vi "Display.vi"(8 "error in":errorcluster, 11 "Custom - Two Button in":refnum<class "Gif - Two Button.lvclass">) -> (0 "error out":errorcluster, 3 "Custom - Two Button out":refnum<class "Gif - Two Button.lvclass">)   [LabVIEW 2021, in "Gif - Two Button.lvclass"]
doc: "This VI will display a custom image to the user along with their message and buttons for pos/neg choice\n\n<b>Code Developed By:</b>\nDaniel Coons\nTechnology Service Corporation\n1983 S Liberty Drive\nBloomington, IN 47403\nPhone: 812 558-7100\ndaniel.coons@tsc.com\nwww.tsc.com/atcs"
uses:
  Gif - Two Button.lvclass
  C:/Program Files/National Instruments/LabVIEW 2024/vi.lib/addons/_TSC/TSC Pop-Up/Popup/Popup.lvclass
  C:/Development/tsc-pop-up-gif/GIF Parent.lvclass
  <vilib>/Utility/miscctls.llb/LVPositionTypeDef.ctl
  Gif - Two Button.lvclass/Gif - Two Button.ctl
  <vilib>/addons/_TSC/TSC Pop-Up/Popup/Popup.lvclass/Popup.ctl
  GIF Parent.lvclass/GIF Parent.ctl
  <vilib>/addons/_TSC/TSC Pop-Up/Popup/Data Member Access/Read Theme.vi
  Read Delays.vi
  Read Gif Images.vi
  <vilib>/addons/_TSC/TSC Pop-Up/Theme/Theme.lvclass
  <vilib>/addons/_TSC/TSC Pop-Up/Popup/Popup.lvclass
  user32.dll
panel:
  in  "closer":bool
  out "header":bool
  in  "n-choice":bool
  in  "y-choice":bool
  out "2D Picture":picture
  out "Message":string
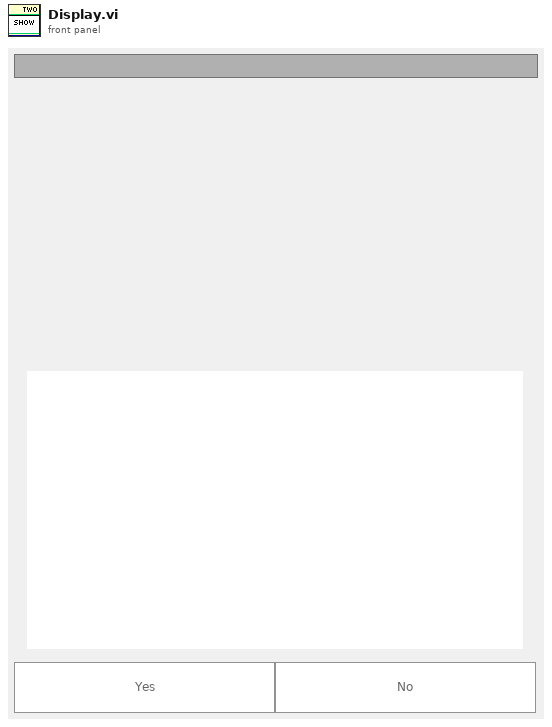
[diagram p1: front panel]
types:
  T1 = typedef "LVPositionTypeDef.ctl" = cluster{"Left":i32, "Top":i32}
  T2 = typedef "LVPoint32TypeDef.ctl" = cluster{"Horizontal":i32, "Vertical":i32}
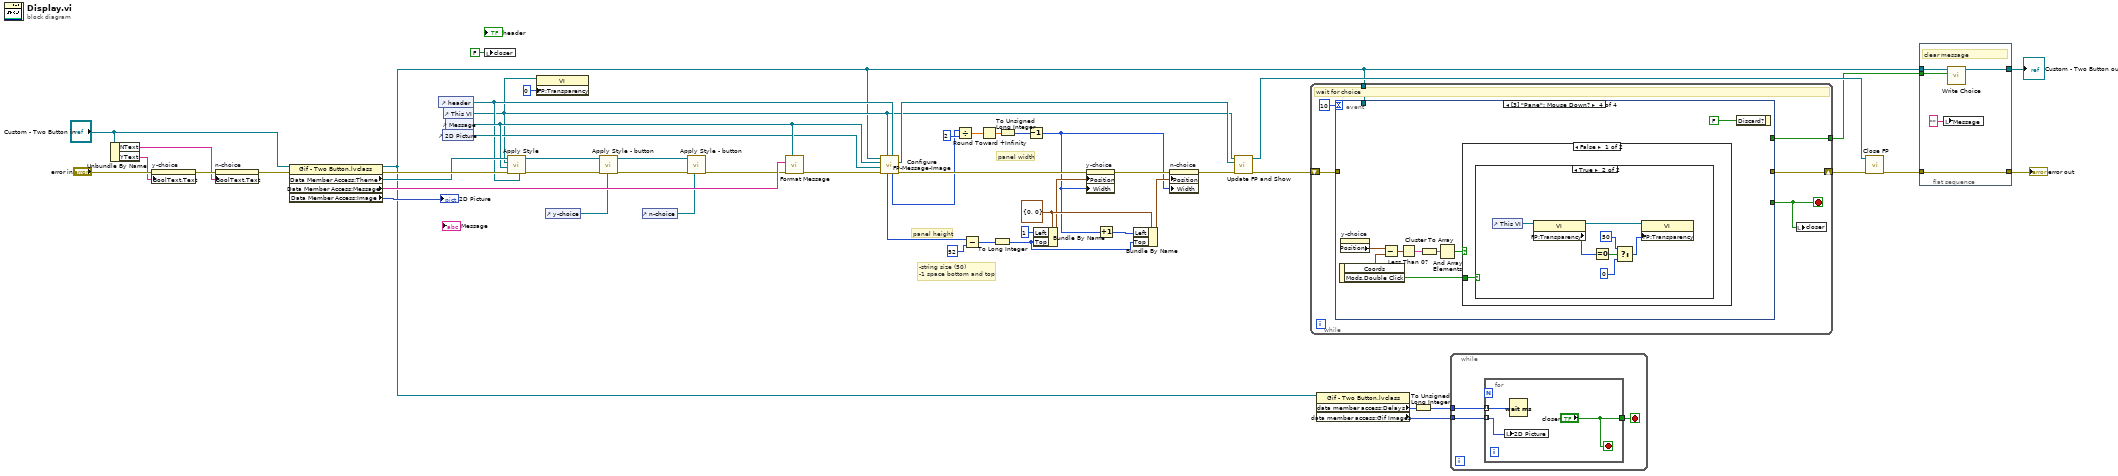
[diagram p0: block diagram]
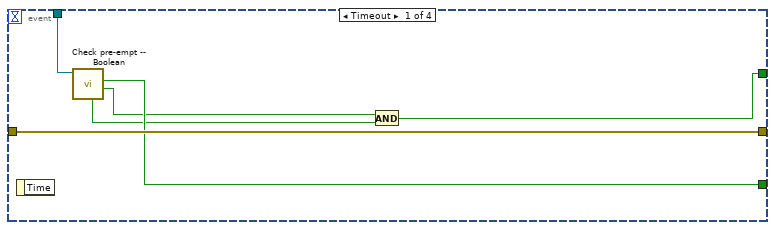
[diagram p2: hidden frame]
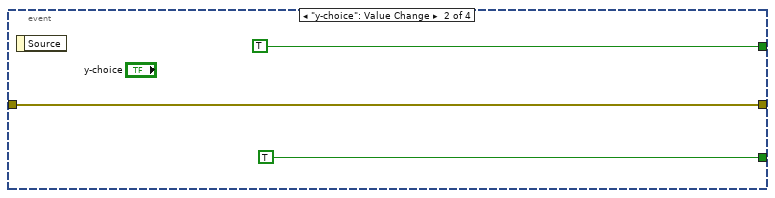
[diagram p3: hidden frame]
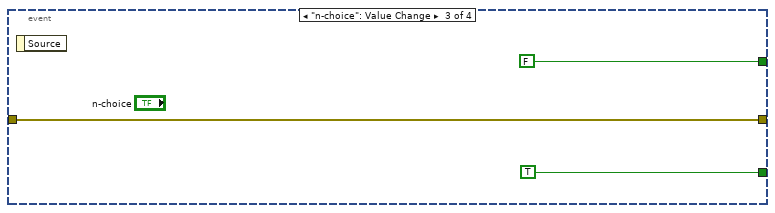
[diagram p4: hidden frame]
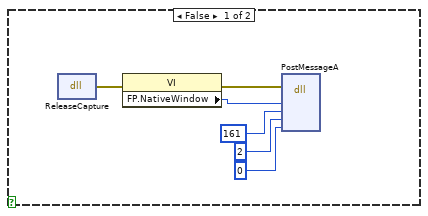
[diagram p5: hidden frame]
diagram:
  w41 = T1 {"Left"=0, "Top"=0} ("Position")
  # "-string size (50)\n-1 space bottom and top"
  # "panel width"
  # "panel height"
  n1 = Unbundle By Name("Custom - Two Button in") -> ("NText"=w43:string, "YText"=w46:string)
  n2 = property on="y-choice" class="Bool"(error in="error in", "BoolText.Text"=w46) -> (error out=w45:errorcluster)  [unwired: 1 in, 1 out]
  n3 = property on="n-choice" class="Bool"(error in=w45, "BoolText.Text"=w43) -> (error out=w44:errorcluster)  [unwired: 1 in, 1 out]
  n4 = property class="Gif - Two Button.lvclass"(reference="Custom - Two Button in", error in=w44) -> (reference out=w1:refnum<class "Gif - Two Button.lvclass">, error out=w28:errorcluster, "Data Member Access:Theme"=w26:refnum<class "Theme.lvclass">, "Data Member Access:Message"=w25:string, "Data Member Access:Image"=→"2D Picture":picture)
  n5 = control-ref of="header"() -> (w14:refnum<vi>)
  n6 = control-ref of="2D Picture"() -> (w15:refnum<vi>)
  n7 = control-ref of="This VI"() -> (w7:refnum<vi>)
  n8 = control-ref of="Message"() -> (w16:refnum<vi>)
  n9 = local write "closer"(FALSE ("closer")) -> ()
  n10 = call <vilib>:"Apply Style.vi"("header ref"=w14, "error in (no error)"=w28, "message ref"=w16, "pop up ref"=w7, "Theme in"=w26) -> ("error out"=w27:errorcluster, "Theme out"=w20:refnum<class "Theme.lvclass">)  [unwired: 5 in]
  n11 = property class="VI"(reference=w7, "FP:Transparency"=u8 0 ("Front Panel Window:Transparency")) -> ()  [unwired: 1 in, 2 out]
  n12 = control-ref of="y-choice"() -> (w21:refnum<vi>)
  n13 = call <vilib>:"Apply Style - button.vi"("button ref"=w21, "error in (no error)"=w27, "Theme in"=w20) -> ("error out"=w23:errorcluster, "Theme out"=w18:refnum<class "Theme.lvclass">)  [unwired: 7 in]
  n14 = control-ref of="n-choice"() -> (w19:refnum<vi>)
  n15 = call <vilib>:"Apply Style - button.vi"("button ref"=w19, "error in (no error)"=w23, "Theme in"=w18) -> ("error out"=w24:errorcluster)  [unwired: 7 in, 1 out]
  n16 = call <vilib>:"Format Message.vi"("formatted string"=w16, "error in"=w24, "String Input"=w25) -> ("error out"=w17:errorcluster)  [unwired: 7 in, 1 out]
  n17 = call <vilib>:"Configure FP-Message-Image.vi"("header ref"=w14, "Pop Up ref"=w7, "error in (no error)"=w17, "Image ref"=w15, "Message ref"=w16, "Popup in"=w1) -> ("error out"=w12:errorcluster, "Panel Ref"=w11:refnum<vi>, "Panel Width"=w10:i32, "Panel Height"=w13:i32)  [unwired: 1 in, 1 out]
  n18 = Divide(x=w10, y=2) -> (x/y=w32:dbl)
  n19 = Subtract(x=w13, y=52 ("value")) -> (x-y=w36:i32)
  n20 = Round Toward +Infinity(x=w32) -> (ceil(x): smallest int >= x=w29:dbl)
  n21 = To Long Integer(number=w36) -> (32bit integer=w39:i32)
  n22 = To Unsigned Long Integer(number=w29) -> (unsigned 32bit integer=w30:u32)
  n23 = Decrement(x=w30) -> (x-1=w8:u32)
  n24 = Bundle By Name(cluster=w41, "Left"=1, "Top"=w39) -> (w37:T1)
  n25 = property on="y-choice" class="Bool"(error in=w12, "Position"=w37, "Width"=w8) -> (error out=w38:errorcluster)  [unwired: 1 in, 1 out]
  n26 = Increment(x=w8) -> (x+1=w9:u32)
  n27 = Bundle By Name(cluster=w41, "Left"=w9, "Top"=w39) -> (w40:T1)
  n28 = property on="n-choice" class="Bool"(error in=w38, "Position"=w40, "Width"=w8) -> (error out=w34:errorcluster)  [unwired: 1 in, 1 out]
  n29 = call <vilib>:"Update FP and Show.vi"("error in (no error)"=w34, "Panel Ref"=w11, "VI in"=w7) -> ("error out"=w49:errorcluster, "VI out"=w50:refnum<vi>)  [unwired: 7 in]
  n30 = while {
    tunnel: [w58] -> w42
    shift-right: [w60] -> w52
    shift-left: w49 -> [w59]
    tunnel: w1 -> [w56]
    stop <- w55 stop-if-true
    # "wait for choice"
    n31 = event shown="[3] \"Pane\": Mouse Down?" {
      selector: _ -> [_ _ _ _]
      dyn-events: _ -> [_ _ _ _]
      timeout: 10 -> [_ _ _ _]
      tunnel: w59 -> [w66 w69 w72 _]
      tunnel: [w66 w69 w72 _] -> w60
      tunnel: [w61 TRUE FALSE _] -> w58
      tunnel: [w64 TRUE TRUE _] -> w55
      tunnel: w56 -> [w65 _ _ _]
      event Timeout {
        n32 = event-data() -> ()  [unwired: 1 in, 1 out]
        n33 = call <vilib>:"Check pre-empt -- Boolean.vi"("_Popup in"=w65) -> ("Value?"=w63:bool, "Pre-empted?"=w64:bool, "Type Match?"=w62:bool)  [unwired: 7 in, 1 out]
        n34 = And(x=w63, y=w62) -> (x .and. y?=w61:bool)
      }
      event "y-choice": Value Change {
        n35 = event-data() -> ()  [unwired: 1 in, 1 out]
      }
      event "n-choice": Value Change {
        n36 = event-data() -> ()  [unwired: 1 in, 1 out]
      }
      event Mouse Down? {
        n37 = event-data() -> ("Coords"=w73:T2, "Mods.Double Click"=w74:bool)  [unwired: 1 in]
        n38 = property on="y-choice" class="Bool"() -> ("Position"=w79:T1)  [unwired: 2 in, 2 out]
        n39 = Subtract(x=w79, y=w73) -> (x-y=w78:T1)
        n40 = Less Than 0?(x=w78) -> (x < 0?=w77:cluster{"Left":bool, "Top":bool})
        n41 = Cluster To Array(cluster=w77) -> (array=w76:bool[])
        n42 = And Array Elements(Boolean array=w76) -> (logical AND=w75:bool)
        n43 = case shown="False" w75 {
          tunnel: w74 -> [w81 _]
          frame False {
            n44 = case shown="True" w81 {
              frame False {
                n45 = dll-call lib="user32.dll" fn="ReleaseCapture"() -> (error out=w85:errorcluster)  [unwired: 4 in, 1 out]
                n46 = property class="VI"(error in=w85) -> (error out=w86:errorcluster, "FP.NativeWindow"=w87:u64)  [unwired: 1 in, 1 out]
                n47 = dll-call lib="user32.dll" fn="PostMessageA"(error in=w86, "hWnd"=w87, "Msg"=161, "wParam"=2, "lParam"=0) -> ()  [unwired: 7 in, 2 out]
              }
              frame True {
                n48 = control-ref of="This VI"() -> (w94:refnum<vi>)
                n49 = property class="VI"(reference=w94) -> (reference out=w92:refnum<vi>, "FP:Transparency"=w93:u8)  [unwired: 1 in, 1 out]
                n50 = Equal To 0?(x=w93) -> (x = 0?=w91:bool)
                n51 = Select(t=u8 50, s=w91, f=u8 0) -> (s? t:f=w90:u8)
                n52 = property class="VI"(reference=w92, "FP:Transparency"=w90) -> ()  [unwired: 1 in, 2 out]
              }
            }
          }
          frame True {
          }
        }
        n53 = event-data("Discard?"=FALSE) -> ()  [unwired: 1 in, 1 out]
      }
    }
    n54 = local write "closer"(w55) -> ()
  }
  n55 = property class="Gif - Two Button.lvclass"(reference=w1) -> ("data member access:Delays"=w5:i32[], "data member access:Gif Images"=w4:picture[])  [unwired: 1 in, 2 out]
  n56 = To Unsigned Long Integer(number=w5) -> (unsigned 32bit integer=w3:u32[])
  n57 = while {
    tunnel: w3 -> [w96]
    tunnel: w4 -> [w95]
    stop <- w97 stop-if-true
    n58 = for {
      tunnel: ["closer"] -> w97
      tunnel: w96 -> [w99] mode=indexing
      tunnel: w95 -> [w98] mode=indexing
      stop <- "closer" stop-if-true
      n59 = local write "2D Picture"(w98) -> ()
      n60 = Wait (ms)(milliseconds to wait=w99) -> ()  [unwired: 1 out]
    }
  }
  n61 = call <vilib>:"Close FP.vi"("error in (no error)"=w52, "VI in"=w50) -> ("error out"=w51:errorcluster)  [unwired: 9 in]
  n62 = flat-sequence {
    tunnel: w51 -> [w105]
    tunnel: [w105] -> w53
    tunnel: w1 -> [w104]
    tunnel: [w102] -> w54
    tunnel: w42 -> [w101]
    frame #0 {
      # "clear message"
      n63 = local write "Message"("" ("Message")) -> ()
      n64 = call-dynamic "Write Choice.vi"("Choice"=w101, "_Popup in"=w104) -> ("_Popup out"=w102:refnum<class "Gif - Two Button.lvclass">)  [unwired: 8 in, 1 out]
    }
  }
  "error out" <- w53
  "Custom - Two Button out" <- w54
